vi "Remove Relays from SwitchActionList Array.vi"(8 "error in (no error)":errorcluster, 9 "Relay Count Subarray [Count>0]":i32[](array[numeric]), 11 "SwitchActionList In":T3 {"RelayAction" items=["CloseRelay"=21, "OpenRelay"=20]}) -> (0 "error out":errorcluster, 1 "Relay Count Subarray [Count>0] Out":i32[](array[numeric]), 3 "SwitchActionList Out":T1[](array[typedef]) {"RelayAction" items=["CloseRelay"=21, "OpenRelay"=20]})   [LabVIEW 2016, in "SLSC Switch.lvlib" / "SLSC Switch.lvclass"]
doc: "Removes Shared Relays from SwitchActionList Array."
uses:
  SLSC Switch.lvclass
  slscsl/SwitchActionsArray.ctl
  slscsl/SwitchAction.ctl
  slscsl/RelayAction.ctl
  slscsl/slscsl.lvclass
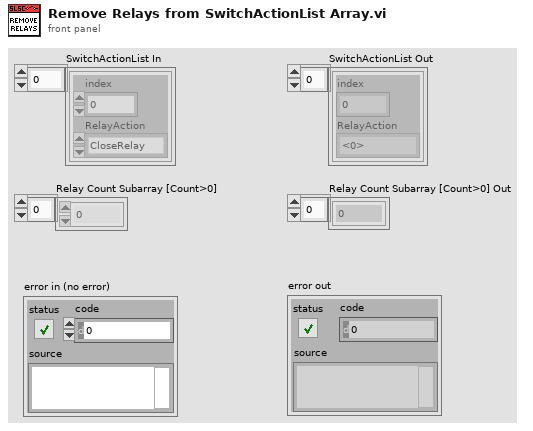
[diagram p1: front panel]
types:
  T1 = typedef "SLSC Switch.lvlib/slscsl.lvclass/SwitchAction.ctl" = cluster{"index":i32, "RelayAction":T2}
  T2 = typedef "SLSC Switch.lvlib/slscsl.lvclass/RelayAction.ctl" = u32
  T3 = typedef "SLSC Switch.lvlib/slscsl.lvclass/SwitchActionsArray.ctl" = T1[]
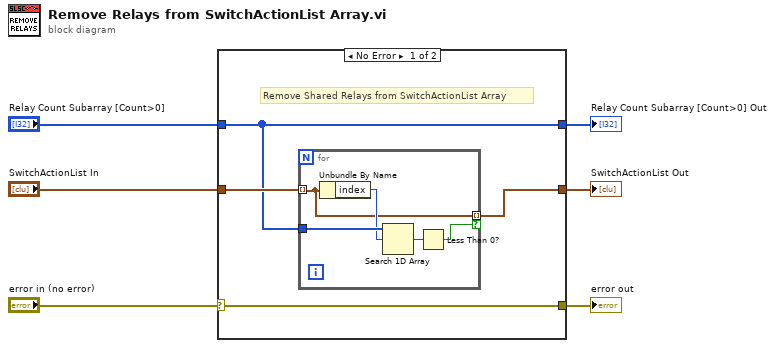
[diagram p0: block diagram]
diagram:
  n1 = case shown="No Error" "error in (no error)" {
    selector: "error in (no error)" -> [w8 w18]
    tunnel: "SwitchActionList In" -> [w10 w17]
    tunnel: [w9 w17] -> w5
    tunnel: "Relay Count Subarray [Count>0]" -> [w7 w16]
    tunnel: [w8 w18] -> w2
    tunnel: [w7 w16] -> w1
    frame No Error {
      # "Remove Shared Relays from SwitchActionList Array"
      n2 = for {
        tunnel: w10 -> [w12] mode=indexing
        tunnel: w7 -> [w15]
        tunnel: [w12] -> w9 mode=indexing if=w11
        n3 = Unbundle By Name(w12) -> ("index"=w14:i32)
        n4 = Search 1D Array(1D array=w15, element=w14) -> (index of element=w13:i32)  [unwired: 1 in]
        n5 = Less Than 0?(x=w13) -> (x < 0?=w11:bool)
      }
    }
    frame Error {
    }
  }
  "SwitchActionList Out" <- w5
  "error out" <- w2
  "Relay Count Subarray [Count>0] Out" <- w1
